vi "Pack Binary Picture.vi"(10 "Threshold":u8, 11 "Image Pixels (U8)":u8[][](array[numeric])) -> (3 "Array":u8[](array[numeric]))   [LabVIEW 2015]
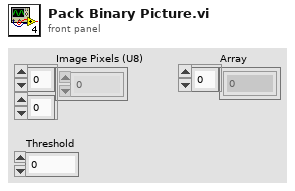
[diagram p1: front panel]
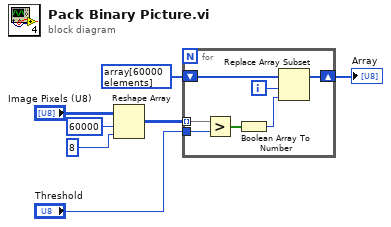
[diagram p0: block diagram]
diagram:
  n1 = Reshape Array("Image Pixels (U8)", 60000 ("dimension size"), 8 ("dimension size")) -> (w7:u8[][])
  n2 = for {
    tunnel: "Threshold" -> [w14]
    shift-right: [w12] -> w3
    shift-left: u8[] array[60000 elements] -> [w13]
    tunnel: w7 -> [w9] mode=indexing
    i -> [w8]
    n3 = Greater?(x=w9, y=w14) -> (0:w11:bool[])
    n4 = Boolean Array To Number(Boolean array=w11) -> (number=w10:u8)
    n5 = Replace Array Subset(array=w13, new element=w10, index=w8) -> (w12:u8[])
  }
  "Array" <- w3
